vi "Position (Reframed) Get.vi"(2 "Z Rescaling":bool, 5 "Frame Properties (m)":T1, 7 "Surface Location (m)":dbl=7.9e-08, 9 "Scaling (mm per pm)":dbl=1.0, 11 "error in (no error)":errorcluster) -> (6 "Reframed Position (m)":cluster{"x (m)":dbl, "y (m)":dbl, "z (m)":dbl} {"z (m)" format="%.1p"; "y (m)" format="%.1p"; "x (m)" format="%.1p"}, 15 "error out":errorcluster)   [LabVIEW 2023, in "Haptic Prog Interface.lvlib"]
doc: "Returns the horizontal xy-position of the haptic pen in nm, and the vertical z-position in mm. The horizontal position depends on the frame origin and frame size.\n\n<b>Z Rescaling:</b> Accepts a booelan. When true, also rescales the vertical position of the pen to nm.\n\n<b>Surface Location:</b> Accepts a double, which is the position in m of the surface.\n\n<b>Scaling:</b> Accepts a double which configures how far the pen must travel in mm for the tip to move a pm.\n\n<b>Frame Properties:</b> Accepts a cluster of two clusters: the first is {x origin (m), y origin (m)}, and the second is {frame width (m), frame height (m)}.\n\n<b>Reframed Position:</b> Returns a cluster of the reframed xyz positions in m."
uses:
  Haptic Prog Interface.lvlib
  Haptic-Programming-Interface/src/x64/Debug/Haptic Programming Interface.dll
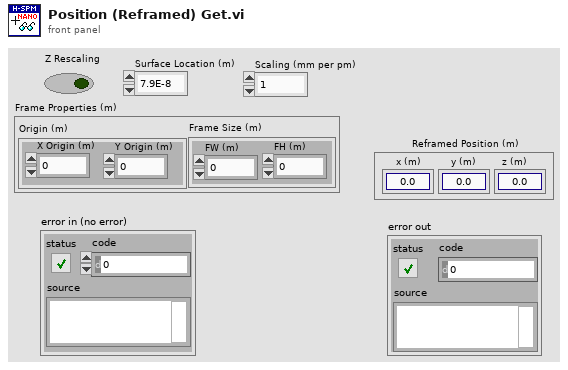
[diagram p1: front panel]
types:
  T1 = cluster{"Origin (m)":cluster{"X Origin (m)":dbl, "Y Origin (m)":dbl}, "Frame Size (m)":cluster{"FW (m)":dbl, "FH (m)":dbl}}
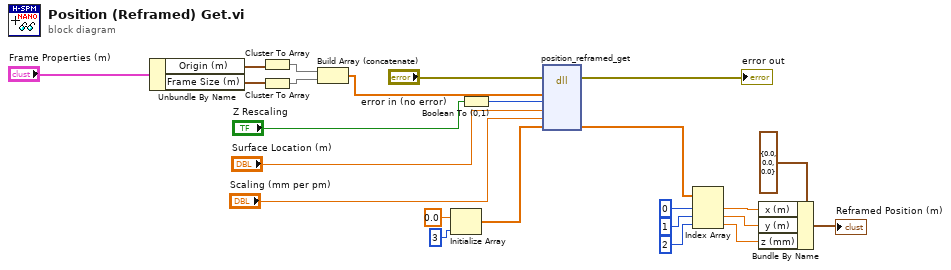
[diagram p0: block diagram]
diagram:
  n1 = Unbundle By Name("Frame Properties (m)") -> ("Origin (m)"=w5:cluster{"X Origin (m)":dbl, "Y Origin (m)":dbl}, "Frame Size (m)"=w4:cluster{"FW (m)":dbl, "FH (m)":dbl})
  n2 = Cluster To Array(cluster=w5) -> (array=w3:dbl[])
  n3 = Cluster To Array(cluster=w4) -> (array=w2:dbl[])
  n4 = Build Array (concatenate)(w3, w2) -> (w1:dbl[])
  n5 = Initialize Array(0.0 ("element"), 3 ("dimension size")) -> (w14:dbl[])
  n6 = Boolean To (0,1)(Boolean="Z Rescaling") -> (0, 1=w10:i16)
  n7 = dll-call lib="C:/Users/cjwel/Documents/GitHub/Haptic-Programming-Interface/src/x64/Debug/Haptic Programming Interface.dll" fn="position_reframed_get"(error in="error in (no error)", "frame_properties"=w1, "zscaling"=w10, "surface_location"="Surface Location (m)", "pos_gain"="Scaling (mm per pm)", "output"=w14) -> (error out=→"error out":errorcluster, "output"=w11:dbl[])  [unwired: 7 in, 1 out]
  n8 = Index Array(array=w11, index #1=0 ("index"), index #2=1 ("index"), index #3=2 ("index")) -> (element #1=w18:dbl, element #2=w17:dbl, element #3=w19:dbl)
  n9 = Bundle By Name(cluster=cluster{"x (m)":dbl, "y (m)":dbl, "z (mm)":dbl} {"x (m)"=0.0, "y (m)"=0.0, "z (mm)"=0.0} ("Position (Reframed)"), "x (m)"=w18, "y (m)"=w17, "z (mm)"=w19) -> (→"Reframed Position (m)":cluster{"x (m)":dbl, "y (m)":dbl, "z (mm)":dbl})
